vi "ctx get device index by id3.vi"(9 "dest_index":u32, 10 "id":u32, 11 "context":u32) -> (1 "dest_index out":u32, 2 "function return":i32, 3 "context out":u32)   [LabVIEW 2019, in "apdm.lvlib"]
doc: "APDM_EXPORT int apdm_ctx_get_device_index_by_id3(apdm_ctx_t context, const uint32_t id, uint32_t *dest_index);"
uses:
  apdm.lvlib
  Lee Lab/CP FES Walking 2018/Code/Working/LabVIEW/apdm.dll
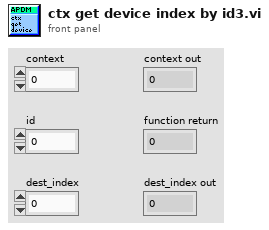
[diagram p1: front panel]
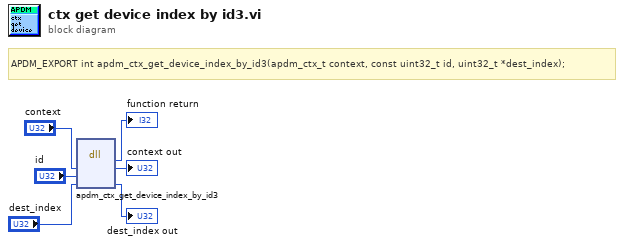
[diagram p0: block diagram]
diagram:
  # "APDM_EXPORT int apdm_ctx_get_device_index_by_id3(apdm_ctx_t context, const uint32_t id, uint32_t *dest_index);"
  n1 = dll-call lib="C:/Users/jfalesi/Dropbox/Lee Lab/CP FES Walking 2018/Code/Working/LabVIEW/apdm.*" fn="apdm_ctx_get_device_index_by_id3"("context"="context", "id"="id", "dest_index"="dest_index") -> (→"function return":i32, "context"=→"context out":u32, "dest_index"=→"dest_index out":u32)  [unwired: 4 in, 2 out]
